vi "SetJointRotation.vi"(8 "error in (no error)":errorcluster, 9 "Rotation (Deg)":dbl, 10 "Joint":T1, 11 "JKI.Robot.SMO":refnum<class "JKI.Robot.SMO.lvclass">) -> (0 "error out":errorcluster, 3 "JKI.Robot.SMO out":refnum<class "JKI.Robot.SMO.lvclass">)   [LabVIEW 2015, in "JKI.Robot.SMO.lvclass"]
doc: "---------------------------------------------------------------\nJKI State Machine Objects™\nhttp://jki.net/state-machine-objects/\nCopyright (C) 2005-2015, JKI <info@jki.net>\nALL RIGHTS RESERVEDJKI State Machine Objects (SMO) 1.0.0.4\nJKI - JKI\nCopyright (c) 2015, JKI"
uses:
  JKI.Robot.SMO.lvclass
  Typedefs/PrivateEvents--JKI.Robot.SMO.SetJointRotation.ctl
  Typedefs/JointType--Enum.ctl
panel:
  # "For instructions on how to use the JKI State Machine Objects, examples and video tutorials, visit:\nhttp://jki.net/state-machine-objects/\n\nJKI State Machine Objects™\nhttp://jki.net/state-machine-objects/\nCopyright (C) 2005-2015, JKI <info@jki.net>\nALL RIGHTS RESERVED"
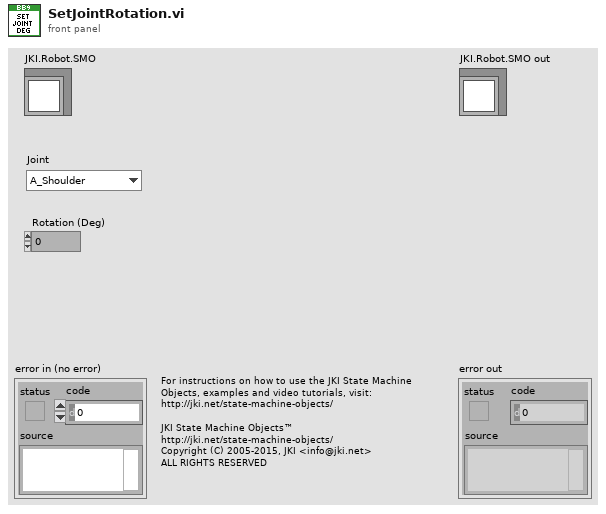
[diagram p1: front panel]
types:
  T1 = typedef "JointType--Enum.ctl" = enum16{"A_Shoulder", "B_Elbow", "C_Wrist", "D_Base"}
  T2 = typedef "JKI.Robot.SMO.lvclass/PrivateEvents--JKI.Robot.SMO.SetJointRotation.ctl" = cluster{"Joint":T1, "Rotation (Deg)":dbl}
  T3 = typedef "JKI.Robot.SMO.lvclass/PrivateData--Ref.ctl" = refnum<data-value>
  T4 = typedef "JKI.Robot.SMO.lvclass/PrivateData--Cluster.ctl" = cluster{"Configuration":T5, "Public Events":T6, "Robot Position":T7, "Private Events":T8}
  T5 = typedef "JKI.Robot.SMO.lvclass/Configuration--Cluster.ctl" = cluster{"Suffix":string}
  T6 = typedef "JKI.Robot.SMO.lvclass/PublicEvents--Cluster.ctl" = cluster{"Data Changed":refnum<user-event>}
  T7 = typedef "RobotPosition--Cluster.ctl" = cluster{"Claw%":dbl, "JointA":dbl, "JointB":dbl, "JointC":dbl, "JointD":dbl}
  T8 = typedef "JKI.Robot.SMO.lvclass/PrivateEvents--Cluster.ctl" = cluster{"SetGrabberPosition":refnum<user-event>, "SetJointRotation":refnum<user-event>}
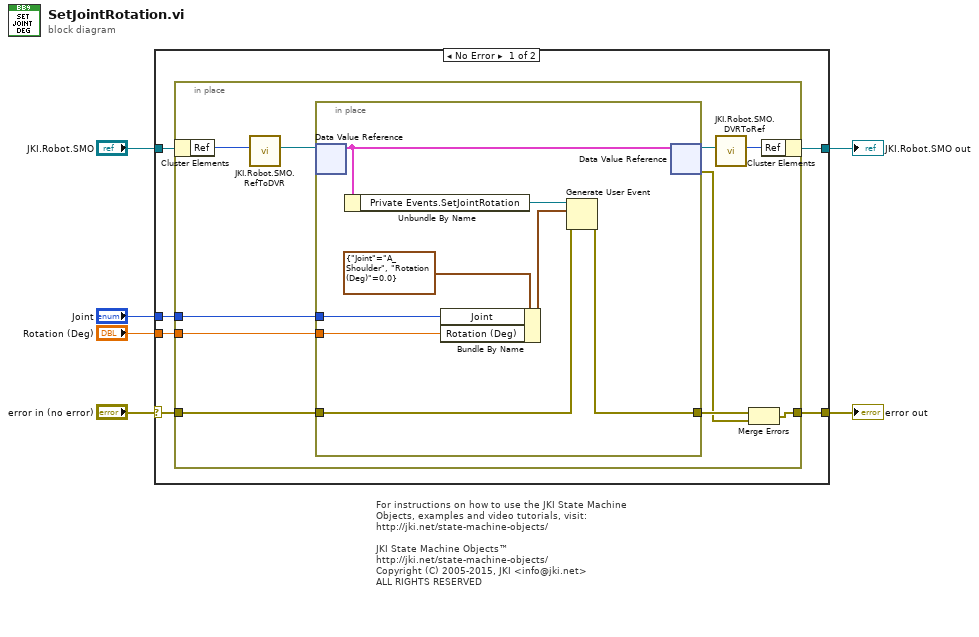
[diagram p0: block diagram]
diagram:
  # "For instructions on how to use the JKI State Machine Objects, examples and video tutorials, visit:\nhttp://jki.net/state-machine-objects/\n\nJKI State Machine Objects™\nhttp://jki.net/state-machine-objects/\nCopyright (C) 2005-2015, JKI <info@jki.net>\nALL RIGHTS RESERVED"
  n1 = case shown="No Error" "error in (no error)" {
    selector: "error in (no error)" -> [w10 w32]
    tunnel: [w9 w32] -> w5
    tunnel: [w11 w31] -> w6
    tunnel: "JKI.Robot.SMO" -> [w12 w31]
    tunnel: "Rotation (Deg)" -> [w8 _]
    tunnel: "Joint" -> [w7 _]
    frame No Error {
      n2 = in-place {
        in-place-border: w10 -> [w22]
        in-place-border: [w19] -> w9
        in-place-border: w8 -> [w14]
        in-place-border: w7 -> [w13]
        n3 = in-place-cluster #1(w12) -> ("Ref"=w18:u32)
        n4 = call "JKI.Robot.SMO.RefToDVR.vi"("Ref"=w18) -> ("Ref"=w16:T3)  [unwired: 10 in]
        n5 = in-place {
          in-place-border: w22 -> [w28]
          in-place-border: [w27] -> w21
          in-place-border: w14 -> [w24]
          in-place-border: w13 -> [w23]
          n6 = in-place-dvr #2(w16) -> (w30:T4)  [unwired: 1 out]
          n7 = Unbundle By Name(w30) -> ("Private Events.SetJointRotation"=w29:refnum<user-event>)
          n8 = Bundle By Name(cluster=T2 {"Joint"=enum."A_Shoulder", "Rotation (Deg)"=0.0} ("SetJointRotation"), "Joint"=w23, "Rotation (Deg)"=w24) -> (w26:T2)
          n9 = Generate User Event(user event=w29, event data cluster=w26, error in=w28) -> (error out=w27:errorcluster)  [unwired: 1 in, 1 out]
          n10 = in-place-dvr #2(w30) -> (w17:T3, w20:errorcluster)
        }
        n11 = call "JKI.Robot.SMO.DVRToRef.vi"("Ref"=w17) -> ("Ref"=w15:u32)  [unwired: 10 in]
        n12 = Merge Errors(w21, w20) -> (w19:errorcluster)
        n13 = in-place-cluster #1("Ref"=w15) -> (w11:refnum<class "JKI.Robot.SMO.lvclass">)
      }
    }
    frame Error {
    }
  }
  "error out" <- w5
  "JKI.Robot.SMO out" <- w6
